vi "Read Message.vi"(6 "timeout in ms [100]":i32=100, 8 "error in (no error)":errorcluster, 10 "index [0]":i32, 11 "RemoteControl.STM in":refnum<class "RemoteControl.STM.lvclass">) -> (0 "error out":errorcluster, 1 "Data":variant, 2 "Command":string, 3 "RemoteControl.STM out":refnum<class "RemoteControl.STM.lvclass">, 4 "ID":string)   [LabVIEW 2019, in "RemoteControl.STM.lvclass"]
uses:
  RemoteControl.STM.lvclass
  C:/Users/patrick/Documents/GitHub/Instrument-Framework/lvsrc/SMOs/RemoteControl/RemoteControl.lvclass
  <vilib>/NI/STM/TCP/TCP Read Options.ctl
  RemoteControl.STM.lvclass/RemoteControl.STM.ctl
  RemoteControl/RemoteControl.lvclass/RemoteControl.ctl
  <vilib>/NI/STM/TCP/Get Connection Reference (TCP).vi
  <vilib>/NI/STM/TCP/Read Message (TCP).vi
  <vilib>/NI/STM/Connection Manager/TCP/TCP Connection Manager.vi
  <vilib>/Utility/error.llb/Error Cluster From Error Code.vi
  <vilib>/ErrorRing/Error Ring.xnode
  <vilib>/NI/STM/NI STM.lvlib
  RemoteControl/RemoteControl.lvclass
  C:/Program Files (x86)/National Instruments/LabVIEW 2019/vi.lib/JKI/JKI SMO/SMO/SMO.lvclass
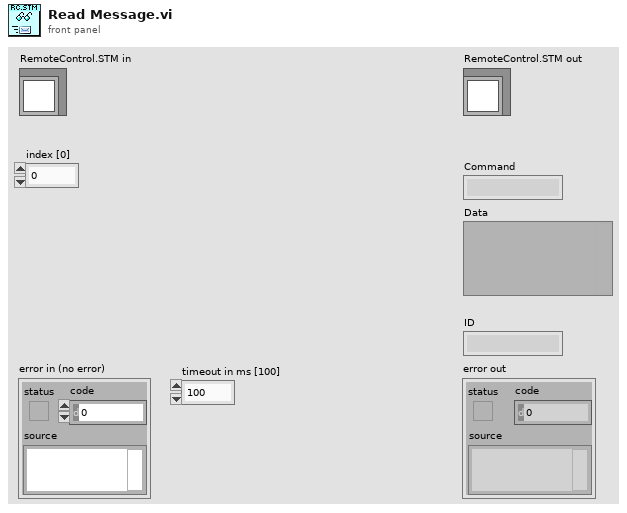
[diagram p1: front panel]
types:
  T1 = typedef "NI STM.lvlib/TCP Read Options.ctl" = cluster{"ignore timeout error":bool, "timeout ms (1000)":i32}
  T2 = typedef "NI STM.lvlib/TCP Connection Info.ctl" = cluster{"connection ID":refnum<k5>, "meta data":T3[]}
  T3 = typedef "NI STM.lvlib/MetaDataElement.ctl" = string
  T4 = typedef "RemoteControl.lvclass/RC Process Type--Enum.ctl" = enum16{"Listener", "Server", "Client"}
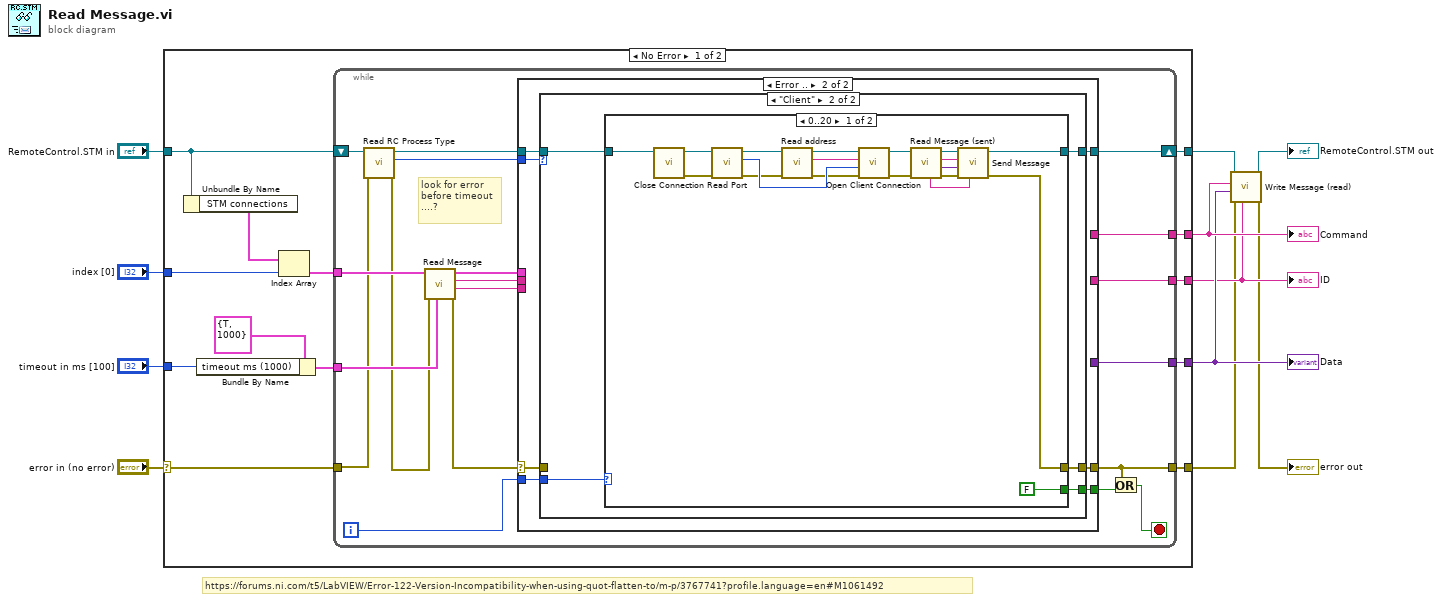
[diagram p0: block diagram]
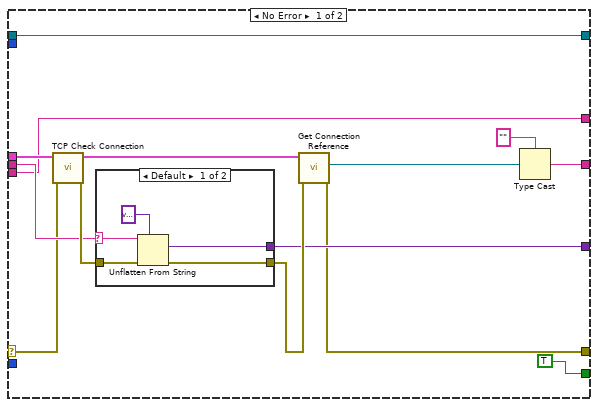
[diagram p2: hidden frame]
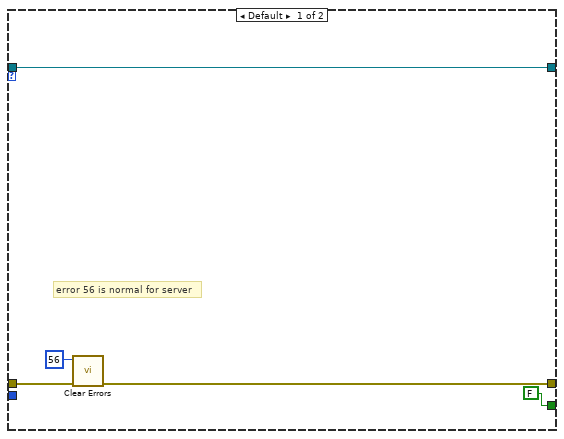
[diagram p4: hidden frame]
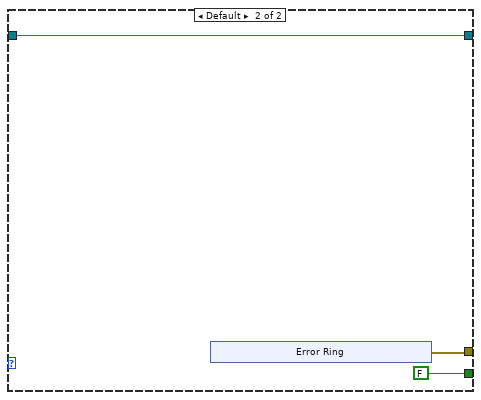
[diagram p5: hidden frame]
diagram:
  # "https://forums.ni.com/t5/LabVIEW/Error-122-Version-Incompatibility-when-using-quot-flatten-to/m-p/3767741?profile.language=en#M1061492"
  n1 = case shown="No Error" "error in (no error)" {
    selector: "error in (no error)" -> [w22 w107]
    tunnel: "timeout in ms [100]" -> [w24 _]
    tunnel: [w14 w107] -> w2
    tunnel: [w19 _] -> w7
    tunnel: [w15 _] -> w6
    tunnel: [w16 _] -> w3
    tunnel: [w13 w108] -> w4
    tunnel: "RemoteControl.STM in" -> [w12 w108]
    tunnel: "index [0]" -> [w20 _]
    frame No Error {
      n2 = Unbundle By Name(w12) -> ("STM connections"=w17:T2[])
      n3 = Bundle By Name(cluster=T1 {"ignore timeout error"=TRUE, "timeout ms (1000)"=1000} ("options"), "timeout ms (1000)"=w24) -> (w18:T1)
      n4 = Index Array(array=w17, index=w20) -> (element=w21:T2)
      n5 = while {
        tunnel: w21 -> [w43]
        tunnel: [w37] -> w19
        tunnel: w18 -> [w40]
        tunnel: [w39] -> w16
        tunnel: [w38] -> w15
        shift-right: [w31] -> w13
        shift-left: w12 -> [w29]
        tunnel: w22 -> [w27]
        tunnel: [w32] -> w14
        i -> [w35]
        stop <- w34 stop-if-true
        # "look for error\nbefore timeout\n....?"
        n6 = call "Read RC Process Type.vi"("error in (no error)"=w27, "RemoteControl in"=w29) -> ("error out"=w26:errorcluster, "RC Process Type"=w30:T4, "RemoteControl out"=w28:refnum<class "RemoteControl.STM.lvclass">)  [unwired: 7 in]
        n7 = call-poly <vilib>:"Read Message.vi"("options"=w40, "error in"=w26, "connection info in"=w43) -> ("error out"=w25:errorcluster, "name"=w36:T3, "data string"=w42:string, "connection info out"=w41:T2)  [unwired: 3 in, 2 out]
        n8 = case shown="Error .." w25 {
          selector: w25 -> [w44 w64]
          tunnel: w42 -> [w46 _]
          tunnel: w41 -> [w55 _]
          tunnel: [w51 _] -> w39
          tunnel: [w50 _] -> w38
          tunnel: [w49 w70] -> w32
          tunnel: [w45 _] -> w37
          tunnel: w36 -> [w45 _]
          tunnel: w35 -> [_ w69]
          tunnel: [TRUE w68] -> w33
          tunnel: [w47 w66] -> w31
          tunnel: w28 -> [w47 w67]
          tunnel: w30 -> [_ w65]
          frame No Error {
            n9 = call <vilib>:"TCP Check Connection.vi"("error in"=w44, "connection in"=w55) -> ("error out"=w53:errorcluster, "connection out"=w54:T2)  [unwired: 7 in, 1 out]
            n10 = case shown="Default" w46 {
              selector: w46 -> [w62 _]
              tunnel: w53 -> [w60 w63]
              tunnel: [w58 w63] -> w52
              tunnel: [w59 _] -> w50
              frame Default {
                n11 = Unflatten From String(type=variant, binary string=w62, error in (no error)=w60) -> (value=w59:variant, error out=w58:errorcluster)  [unwired: 2 in, 1 out]
              }
              frame "" {
              }
            }
            n12 = call-poly <vilib>:"Get Connection Reference.vi"("error in"=w52, "connection info in"=w54) -> ("error out"=w49:errorcluster, "connection ID out"=w57:refnum<k5>)  [unwired: 7 in, 1 out]
            n13 = Type Cast(type="", x=w57) -> (*(type *) &x=w51:string)
          }
          frame Error {
            n14 = case shown="\"Client\"" w65 {
              tunnel: [w71 w80] -> w70
              tunnel: w69 -> [_ w76]
              tunnel: [FALSE w79] -> w68
              tunnel: w67 -> [w74 w78]
              tunnel: [w74 w77] -> w66
              tunnel: w64 -> [w73 _]
              frame Default {
                # "error 56 is normal for server"
                n15 = call <vilib>:"Clear Errors.vi"("error in (no error)"=w73, "specific error code to clear (0: all)"=56) -> ("error out"=w71:errorcluster)  [unwired: 4 in, 1 out]
              }
              frame "Client" {
                n16 = case shown="0..20" w76 {
                  tunnel: [w97 w101] -> w80
                  tunnel: [FALSE FALSE] -> w79
                  tunnel: w78 -> [w81 w100]
                  tunnel: [w98 w100] -> w77
                  frame 0..20 {
                    n17 = call-dynamic "Close Connection.vi"("RemoteControl.STM in"=w81) -> ("error out"=w83:errorcluster, "RemoteControl.STM out"=w89:refnum<class "RemoteControl.STM.lvclass">)  [unwired: 9 in]
                    n18 = call-dynamic "Read Port.vi"("error in (no error)"=w83, "RemoteControl in"=w89) -> ("error out"=w84:errorcluster, "Port"=w85:u16, "RemoteControl out"=w88:refnum<class "RemoteControl.STM.lvclass">)  [unwired: 7 in]
                    n19 = call-dynamic "Read address.vi"("error in (no error)"=w84, "RemoteControl in"=w88) -> ("error out"=w82:errorcluster, "address"=w86:string, "RemoteControl out"=w87:refnum<class "RemoteControl.STM.lvclass">)  [unwired: 7 in]
                    n20 = call-dynamic "Open Client Connection.vi"("error in (no error)"=w82, "Port"=w85, "address"=w86, "RemoteControl.STM in"=w87) -> ("error out"=w90:errorcluster, "RemoteControl.STM out"=w91:refnum<class "RemoteControl.STM.lvclass">)  [unwired: 6 in]
                    n21 = call "Read Message (sent).vi"("error in (no error)"=w90, "RemoteControl in"=w91) -> ("error out"=w93:errorcluster, "Data (Sent)"=w94:variant, "Command (Sent)"=w95:string, "RemoteControl out"=w96:refnum<class "RemoteControl.STM.lvclass">, "ID (Sent)"=w92:string)  [unwired: 5 in]
                    n22 = call-dynamic "Send Message.vi"("ID"=w92, "error in (no error)"=w93, "Data"=w94, "Command"=w95, "RemoteControl.STM in"=w96) -> ("error out"=w97:errorcluster, "RemoteControl.STM out"=w98:refnum<class "RemoteControl.STM.lvclass">)  [unwired: 4 in, 1 out]
                  }
                  frame Default {
                    n23 = xnode "Error Ring"() -> ("error out"=w101:errorcluster)
                  }
                }
              }
            }
          }
        }
        n24 = Or(x=w32, y=w33) -> (x .or. y?=w34:bool)
      }
    }
    frame Error {
    }
  }
  "ID" <- w3
  "Data" <- w6
  "Command" <- w7
  n25 = call "Write Message (read).vi"("ID (Read)"=w3, "error in (no error)"=w2, "Data (Read)"=w6, "Command (Read)"=w7, "RemoteControl in"=w4) -> ("error out"=→"error out":errorcluster, "RemoteControl out"=→"RemoteControl.STM out":refnum<class "RemoteControl.STM.lvclass">)  [unwired: 5 in]
